vi "ke37xx Measure.vi"(0 "VISA Resource Name":refnum<visa-resource-name>, 5 "Buffer Name":string, 7 "Measure Count (1)":u32=1, 9 "Time Stamps (0: None)":T1(ring), 11 "error in (no error)":errorcluster) -> (4 "VISA Resource Name Out":refnum<visa-resource-name>, 6 "Reading":dbl format="%#_6e", 8 "Seconds":u32, 10 "Fractional Seconds":dbl, 15 "error out":errorcluster)   [LabVIEW 2009, in "Keithley 3700 Series.lvlib"]
doc: "This VI allows you to perform both single-point and multi-point measurements. The measurement is performed immediately, without the use of the trigger model. In the case of multi-point measurements, the readings taken are stored in a measurement buffer."
uses:
  <instrlib>/Keithley 3706/Keithley 3700 Series.lvlib
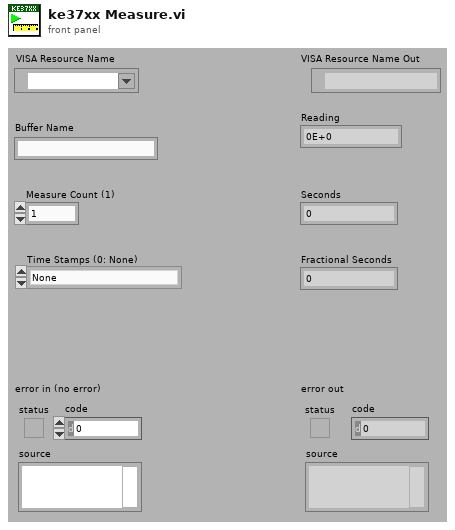
[diagram p1: front panel]
types:
  T1 = enum16{"None", "Include UTC Time Stamps", "Include 1588 Time Stamps"}
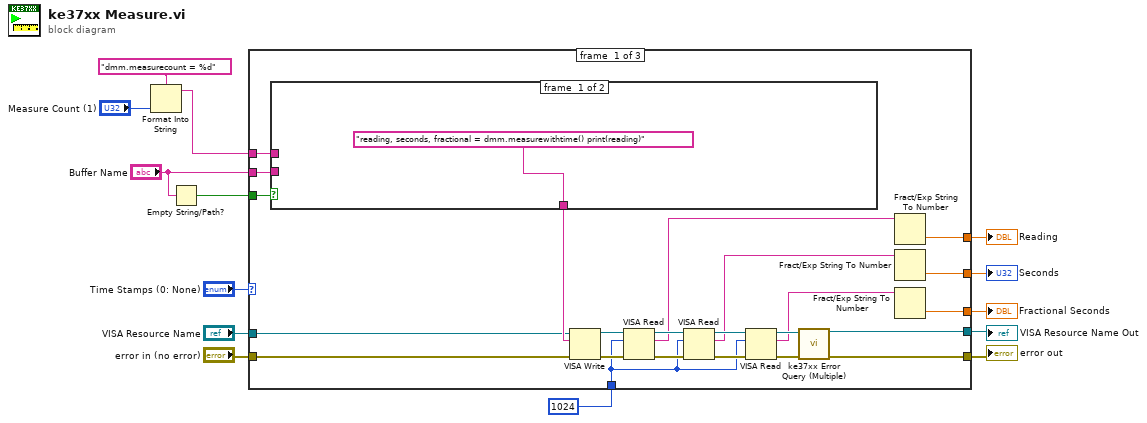
[diagram p0: block diagram]
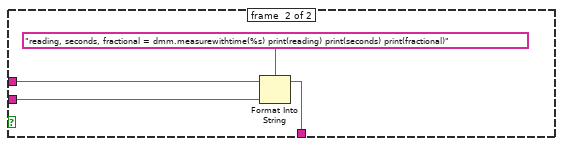
[diagram p2: hidden frame]
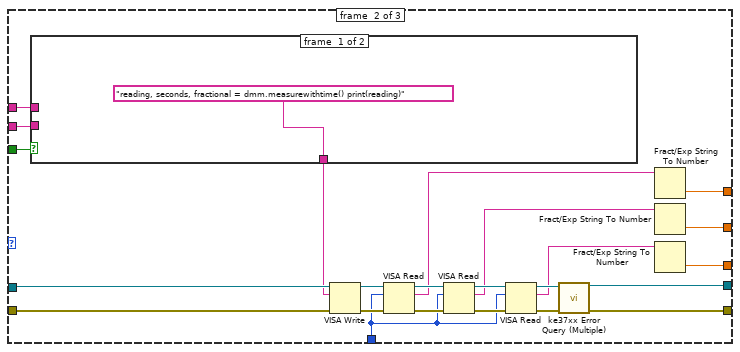
[diagram p3: hidden frame]
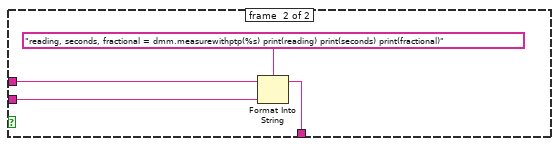
[diagram p4: hidden frame]
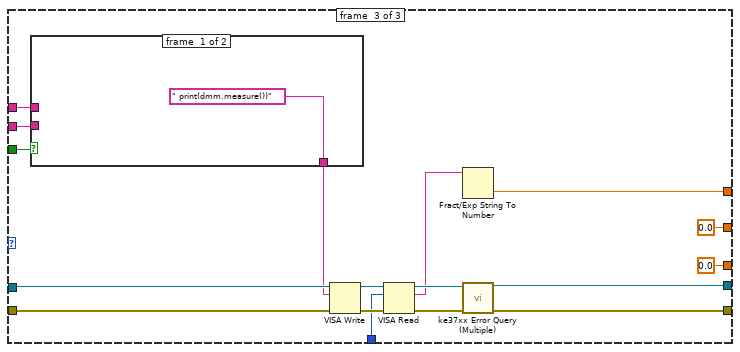
[diagram p5: hidden frame]
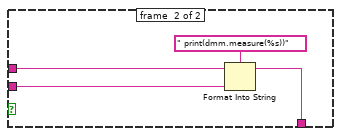
[diagram p6: hidden frame]
diagram:
  n1 = Format Into String(format string="dmm.measurecount = %d", "Measure Count (1)") -> (resulting string=w10:string)  [unwired: 2 in, 1 out]
  n2 = Empty String/Path?(string/path="Buffer Name") -> (empty?=w9:bool)
  n3 = case shown="\"None\"" "Time Stamps (0: None)" {
    tunnel: [w36 w63 w86] -> w14
    tunnel: [w35 w62 w85] -> w13
    tunnel: u32 1024 -> [w21 w48 w79]
    tunnel: w10 -> [w31 w58 w78]
    tunnel: w9 -> [w30 w57 w77]
    tunnel: "Buffer Name" -> [w29 w56 w76]
    tunnel: [w27 w54 w74] -> w7
    tunnel: [w20 w47 0.0] -> w5
    tunnel: [w19 w46 0.0] -> w4
    tunnel: "VISA Resource Name" -> [w15 w65 w87]
    tunnel: "error in (no error)" -> [w16 w43 w71]
    frame #0 {
      n4 = case shown="False" w30 {
        tunnel: ["reading, seconds, fractional = dmm.measurewithtime() print(reading)" w41] -> w34
        tunnel: w31 -> [_ w40]
        tunnel: w29 -> [_ w39]
        frame #0 {
        }
        frame #1 {
          n5 = Format Into String(format string="reading, seconds, fractional = dmm.measurewithtime(%s) print(reading) print(seconds) print(fractional)", initial string=w40, w39) -> (resulting string=w41:string)  [unwired: 1 in, 1 out]
        }
      }
      n6 = VISA Write(VISA resource name=w15, write buffer=w34, error in (no error)=w16) -> (VISA resource name out=w33:refnum<visa-resource-name>, error out=w32:errorcluster)  [unwired: 1 out]
      n7 = VISA Read(VISA resource name=w33, byte count=w21, error in (no error)=w32) -> (VISA resource name out=w37:refnum<visa-resource-name>, read buffer=w28:string, error out=w24:errorcluster)  [unwired: 1 out]
      n8 = VISA Read(VISA resource name=w37, byte count=w21, error in (no error)=w24) -> (VISA resource name out=w26:refnum<visa-resource-name>, read buffer=w18:string, error out=w23:errorcluster)  [unwired: 1 out]
      n9 = VISA Read(VISA resource name=w26, byte count=w21, error in (no error)=w23) -> (VISA resource name out=w25:refnum<visa-resource-name>, read buffer=w17:string, error out=w22:errorcluster)  [unwired: 1 out]
      n10 = call <instrlib>:"ke37xx Error Query (Multiple).vi"("VISA resource name"=w25, "error in (no error)"=w22) -> ("VISA resource name out"=w36:refnum<visa-resource-name>, "error out"=w35:errorcluster)  [unwired: 12 out]
      n11 = Fract/Exp String To Number(string=w28) -> (number=w27:dbl)  [unwired: 4 out]
      n12 = Fract/Exp String To Number(string=w18) -> (number=w20:dbl)  [unwired: 4 out]
      n13 = Fract/Exp String To Number(string=w17) -> (number=w19:dbl)  [unwired: 4 out]
    }
    frame #1 {
      n14 = case shown="False" w57 {
        tunnel: ["reading, seconds, fractional = dmm.measurewithtime() print(reading)" w69] -> w61
        tunnel: w58 -> [_ w68]
        tunnel: w56 -> [_ w67]
        frame #0 {
        }
        frame #1 {
          n15 = Format Into String(format string="reading, seconds, fractional = dmm.measurewithptp(%s) print(reading) print(seconds) print(fractional)", initial string=w68, w67) -> (resulting string=w69:string)  [unwired: 1 in, 1 out]
        }
      }
      n16 = VISA Write(VISA resource name=w65, write buffer=w61, error in (no error)=w43) -> (VISA resource name out=w60:refnum<visa-resource-name>, error out=w59:errorcluster)  [unwired: 1 out]
      n17 = VISA Read(VISA resource name=w60, byte count=w48, error in (no error)=w59) -> (VISA resource name out=w64:refnum<visa-resource-name>, read buffer=w55:string, error out=w51:errorcluster)  [unwired: 1 out]
      n18 = VISA Read(VISA resource name=w64, byte count=w48, error in (no error)=w51) -> (VISA resource name out=w53:refnum<visa-resource-name>, read buffer=w45:string, error out=w50:errorcluster)  [unwired: 1 out]
      n19 = VISA Read(VISA resource name=w53, byte count=w48, error in (no error)=w50) -> (VISA resource name out=w52:refnum<visa-resource-name>, read buffer=w44:string, error out=w49:errorcluster)  [unwired: 1 out]
      n20 = call <instrlib>:"ke37xx Error Query (Multiple).vi"("VISA resource name"=w52, "error in (no error)"=w49) -> ("VISA resource name out"=w63:refnum<visa-resource-name>, "error out"=w62:errorcluster)  [unwired: 12 out]
      n21 = Fract/Exp String To Number(string=w55) -> (number=w54:dbl)  [unwired: 4 out]
      n22 = Fract/Exp String To Number(string=w45) -> (number=w47:dbl)  [unwired: 4 out]
      n23 = Fract/Exp String To Number(string=w44) -> (number=w46:dbl)  [unwired: 4 out]
    }
    frame #2 {
      n24 = case shown="False" w77 {
        tunnel: [" print(dmm.measure())" w91] -> w84
        tunnel: w78 -> [_ w90]
        tunnel: w76 -> [_ w89]
        frame #0 {
        }
        frame #1 {
          n25 = Format Into String(format string=" print(dmm.measure(%s))", initial string=w90, w89) -> (resulting string=w91:string)  [unwired: 1 in, 1 out]
        }
      }
      n26 = VISA Write(VISA resource name=w87, write buffer=w84, error in (no error)=w71) -> (VISA resource name out=w83:refnum<visa-resource-name>, error out=w81:errorcluster)  [unwired: 1 out]
      n27 = VISA Read(VISA resource name=w83, byte count=w79, error in (no error)=w81) -> (VISA resource name out=w82:refnum<visa-resource-name>, read buffer=w75:string, error out=w80:errorcluster)  [unwired: 1 out]
      n28 = Fract/Exp String To Number(string=w75) -> (number=w74:dbl)  [unwired: 4 out]
      n29 = call <instrlib>:"ke37xx Error Query (Multiple).vi"("VISA resource name"=w82, "error in (no error)"=w80) -> ("VISA resource name out"=w86:refnum<visa-resource-name>, "error out"=w85:errorcluster)  [unwired: 12 out]
    }
  }
  "VISA Resource Name Out" <- w14
  "error out" <- w13
  "Reading" <- w7
  "Fractional Seconds" <- w4
  "Seconds" <- w5
